vi "side_features.vi"() -> ()   [LabVIEW 2015]
uses:
  <vilib>/Analysis/baseanly.llb/Mean (DBL).vi
  <vilib>/Utility/file.llb/Read Delimited Spreadsheet (string).vi
  <vilib>/Utility/file.llb/Write Delimited Spreadsheet (string).vi
  <vilib>/vision/NI_Vision_Development_Module.lvlib
  PlantType.dll
  TotalContoursConvexHull.dll
  2-top_features_oilseed/HistProperty.dll
  <vilib>/Analysis/NI_AALBase.lvlib
panel:
  out "savePath":path
  out "appended array":string[](array[string])
  out "im_width":i32
  out "im_height":i32
  in  "Date Path":path=path "H:/3-side_features_oilseed/rape_test/path.txt"
  out "Current Path":path
  out "Current Number":string
  out "Rotated Image":T1(plugin-control)
  out "HistStat_whole":dbl[](array[numeric])
  out "PAR (perimeter-to-area ratio)":dbl
  out "SFD":sgl
  out "BW (minimum circumscribed box width)":dbl
  out "BH (minimum circumscribed box height)":dbl
  out "TPA (Total projective area)":dbl
  out "R (Rectangularity)":dbl
  out "IFD":sgl
  out "Hull area":dbl
  out "AC (Area Convexity)":dbl
  out "HWR":dbl
  in  "ROI_flower":T2={"Top"=0, "im_height"=1450, "L_left"=0, "im_width"=1680}
  out "NB (Number of blanchs)":i32
  out "FPAR (Flower perimeter-to-area ratio)":dbl
  out "FSFD":sgl
  out "FBW (Flower minimum circumscribed box width)":dbl
  out "FBH (Flower minimum circumscribed box height)":dbl
  out "YPA (Yellow projective area)":dbl
  out "FR (Flower rectangularity)":dbl
  out "FIFD":sgl
  out "FAC (Flower area Convexity)":dbl
  out "HistStat_flower":dbl[](array[numeric])
  in  "ROI_whole":T2={"Top"=90, "im_height"=1970, "L_left"=300, "im_width"=1450}
  out "FHWR":dbl
  out "GPA (Green projective area)":dbl
  out "GPAR (Green / Total)":dbl
  out "YPAR (Yellow / Total)":dbl
  out "Flower Hull Image":T1(plugin-control)
  out "Flower Hull Area":dbl
  out "Cropped Image":T1(plugin-control)
  out "Binary Image":T1(plugin-control)
  out "rgb Hull Image":T1(plugin-control)
  out "Flower Image (RGB)":T1(plugin-control)
  out "Flower Image (Label)":T1(plugin-control)
  out "PD1-6":sgl[](array[numeric])
  out "f array":dbl[](array[numeric])
  out "Combined Image":T1(plugin-control)
  out "Image Path":path
  in  "Image Main Path":path=path "H:/3-side_features_oilseed/rape_test"
  # "Digital evaluation software for oilseed rape phenotype-related traits (side-view) v1.0"
  # "测量数据"
  # "Whole plant"
  # "均值"
  # "标准差"
  # "平滑度"
  # "三阶矩"
  # "一致性"
  # "熵"
  # "Flower"
  # "Ratio"
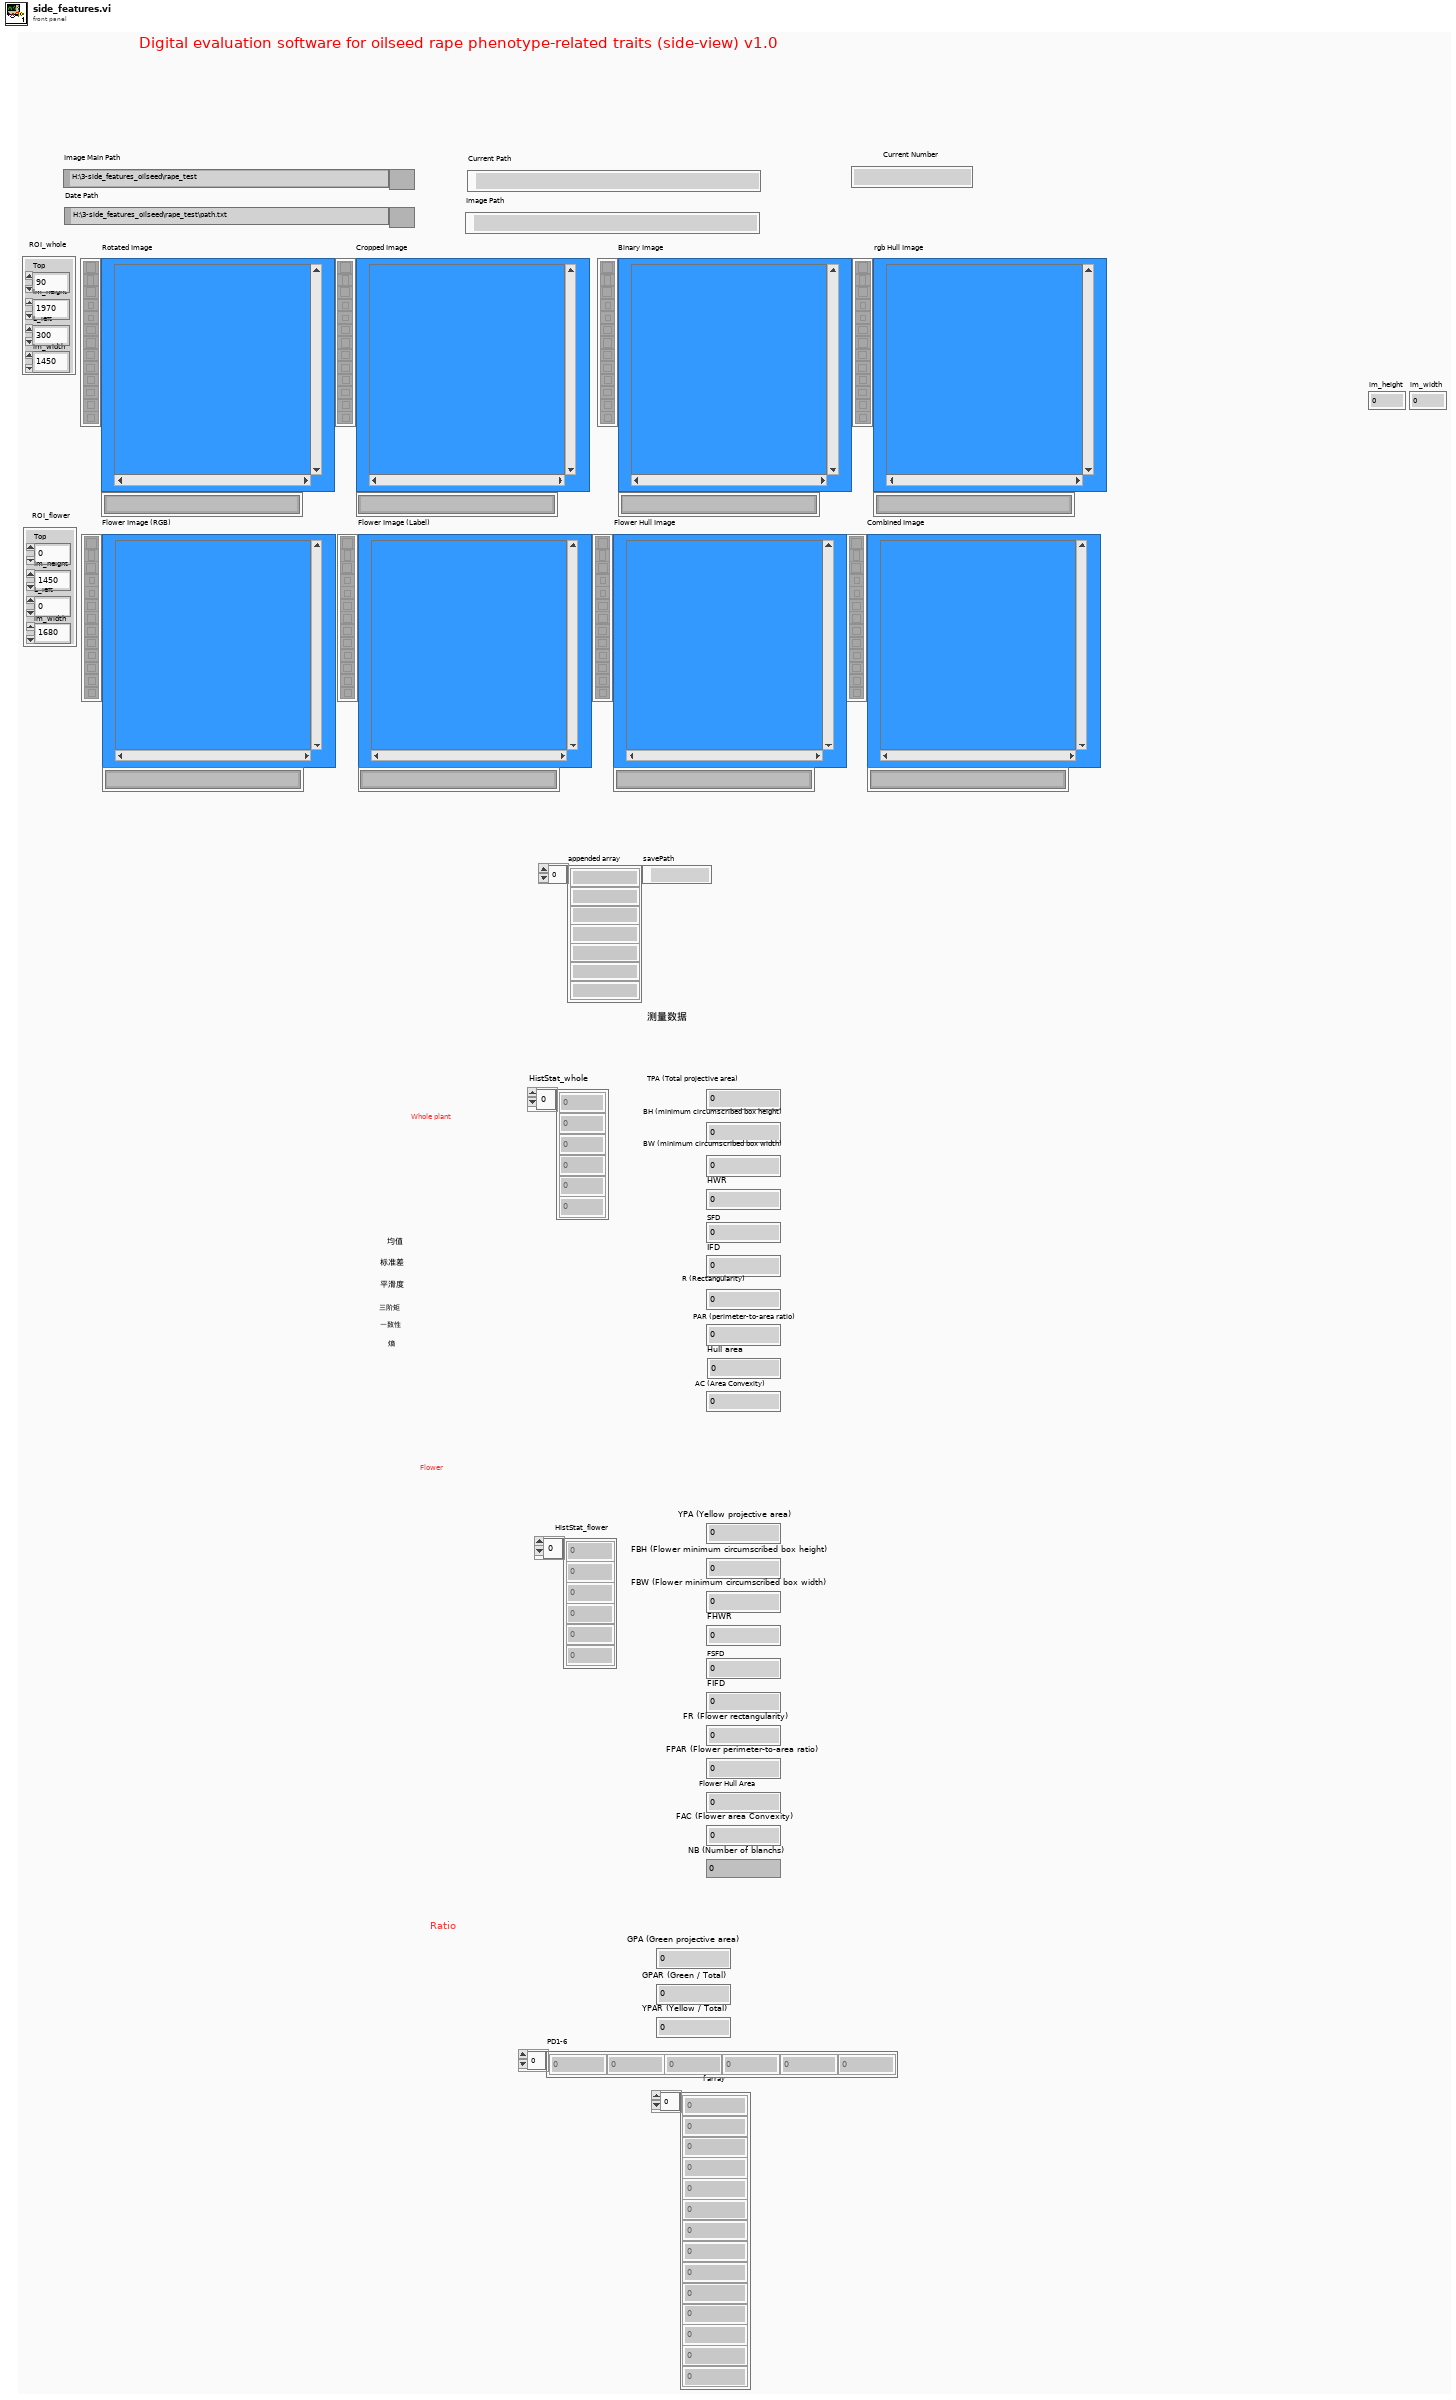
[diagram p1: front panel]
types:
  T1 = typedef "IMAQ Image.ctl" = refnum<image>
  T2 = cluster{"Top":i32, "im_height":i32, "L_left":i32, "im_width":i32}
  T3 = typedef "Image Type" = u32
  T4 = typedef "Particle Parameters" = i32
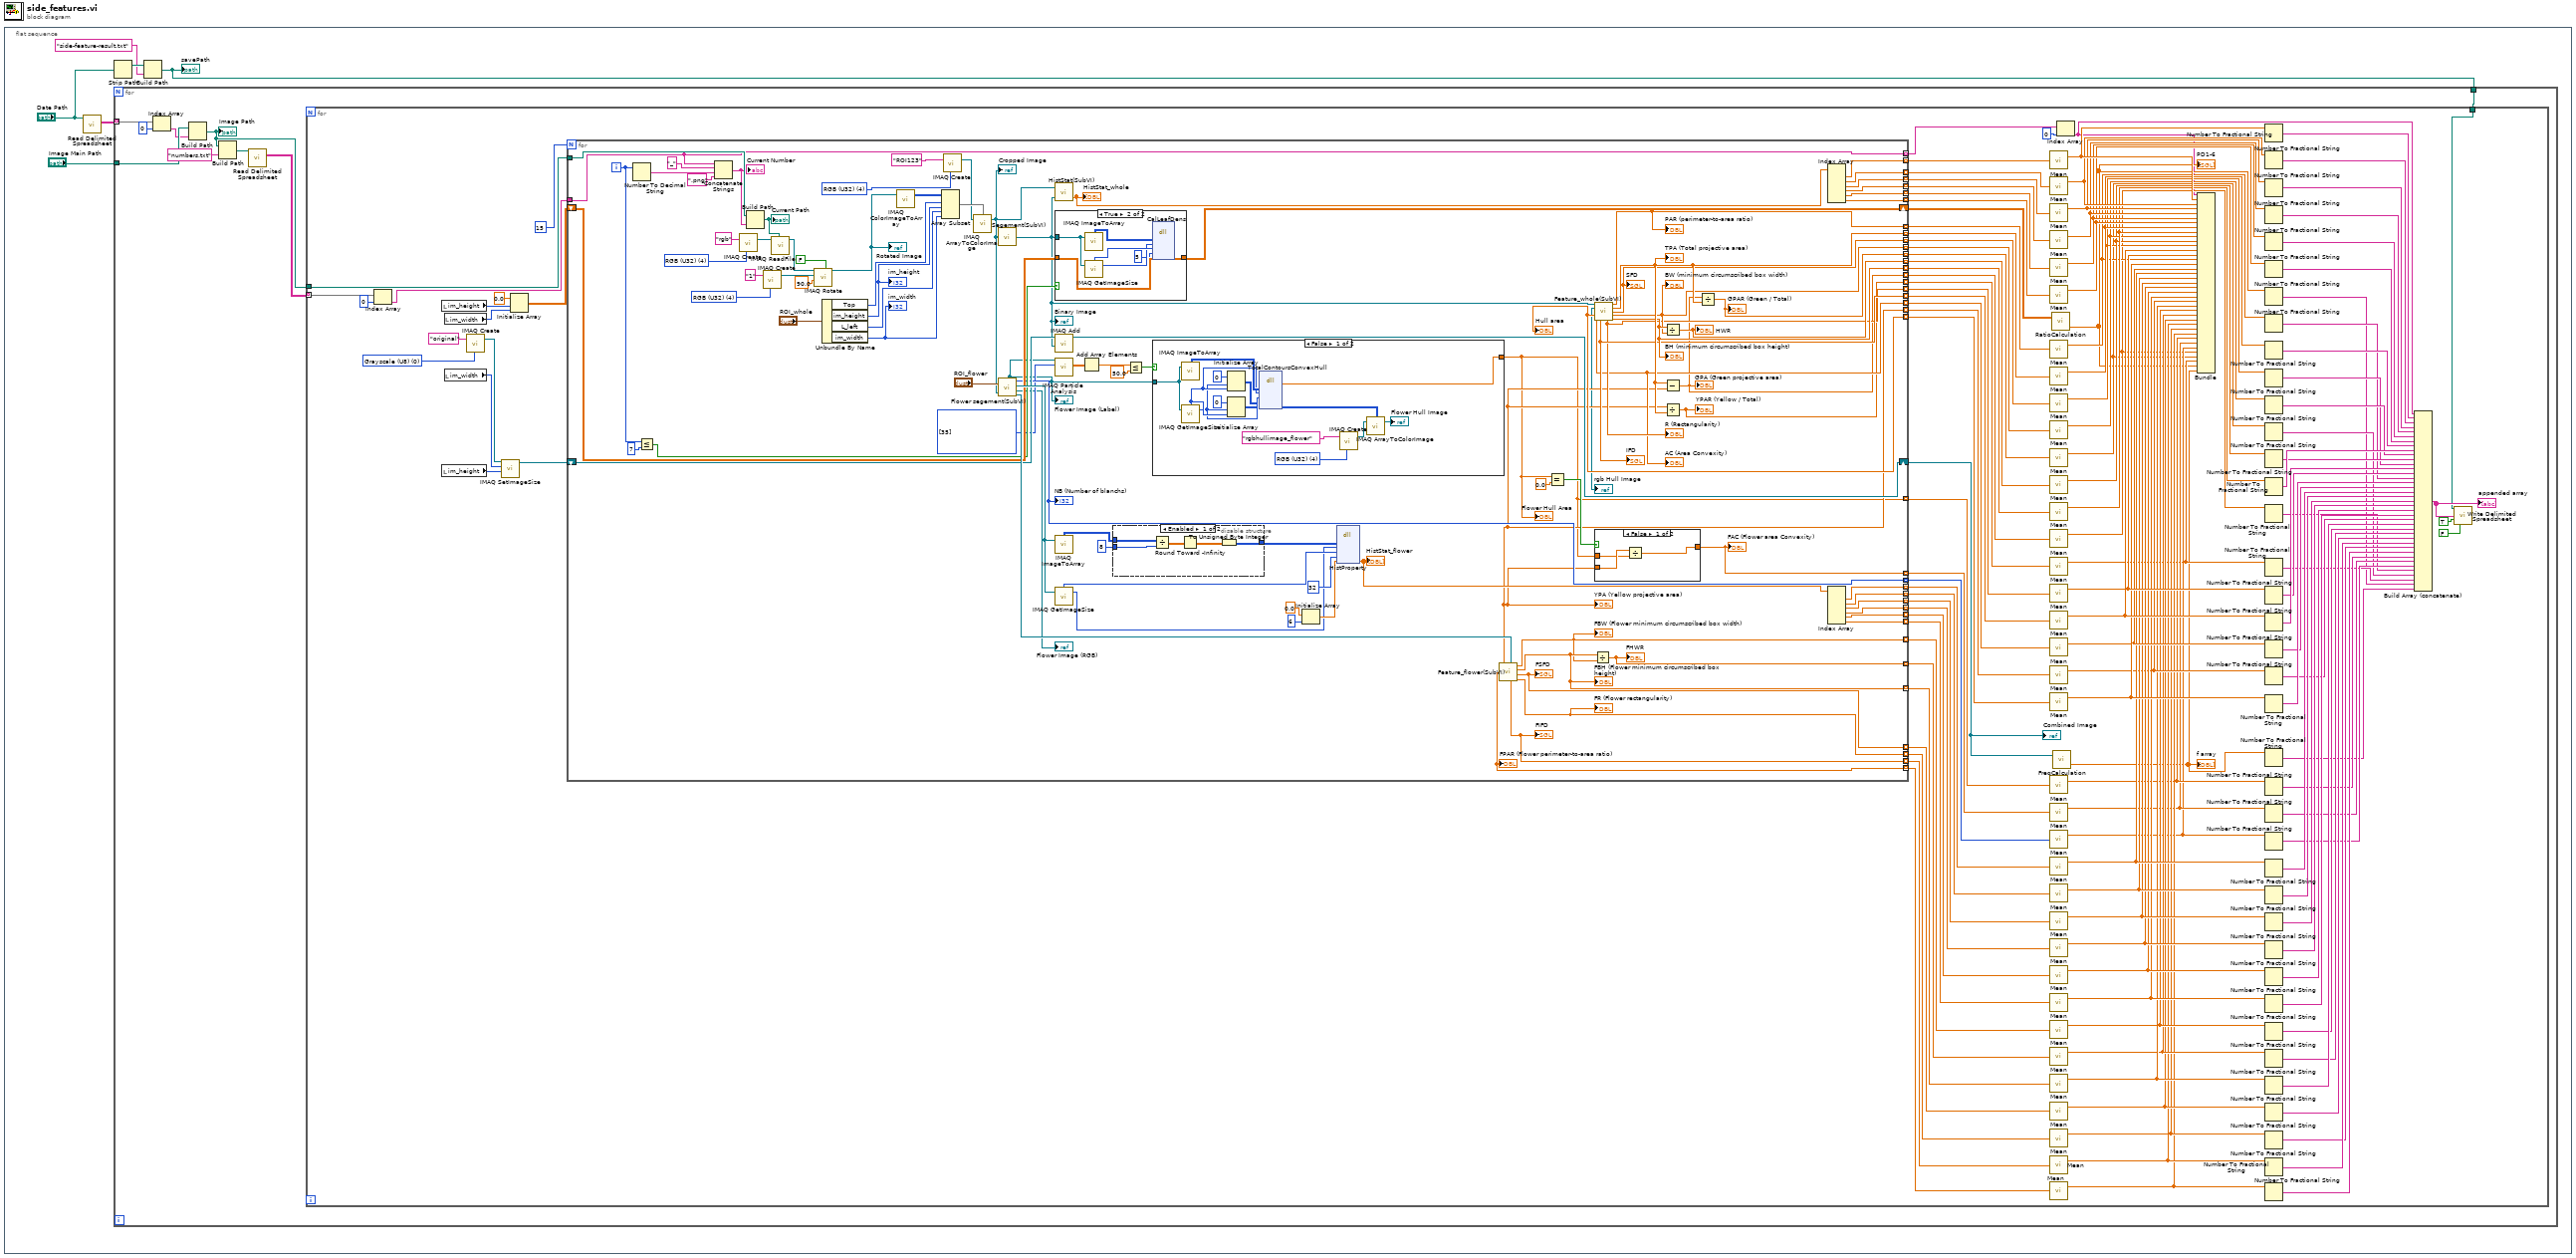
[diagram p0: block diagram]
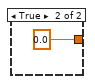
[diagram p2: hidden frame]
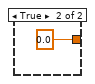
[diagram p3: hidden frame]
diagram:
  n1 = flat-sequence {
    frame #0 {
      n2 = call-poly <vilib>:"Read Delimited Spreadsheet.vi"("file path (dialog if empty)"="Date Path") -> ("all rows"=w5:string[][])  [unwired: 9 in, 5 out]
      n3 = Strip Path(path="Date Path") -> (stripped path=w3:path)  [unwired: 1 out]
      n4 = Build Path(base path=w3, name or relative path="side-feature-result.txt") -> (appended path=w1:path)
      "savePath" <- w1
      n5 = for {
        tunnel: "Image Main Path" -> [w15]
        tunnel: w5 -> [w13] mode=indexing
        tunnel: w1 -> [w7]
        n6 = Index Array(array=w13, index=0) -> (element=w9:string)
        n7 = Build Path(base path=w15, name or relative path=w9) -> (appended path=w10:path)
        "Image Path" <- w10
        n8 = Build Path(base path=w10, name or relative path="numbers.txt") -> (appended path=w11:path)
        n9 = call-poly <vilib>:"Read Delimited Spreadsheet.vi"("file path (dialog if empty)"=w11) -> ("all rows"=w8:string[][])  [unwired: 9 in, 5 out]
        n10 = for {
          tunnel: w10 -> [w149]
          tunnel: w8 -> [w150] mode=indexing
          tunnel: w7 -> [w16]
          w141 = T3 0 items=["Grayscale (U8)", "Grayscale (I16)", "Grayscale (SGL)", "Complex (CSG)", "RGB (U32)", "HSL (U32)", "RGB (U64)", "Grayscale (U16)"] ("Image Type")
          n11 = Index Array(array=w150, index=0) -> (element=w148:string)
          n12 = local read "im_height"() -> (w100:i32)
          n13 = local read "im_height"() -> (w99:i32)
          n14 = local read "im_width"() -> (w98:i32)
          n15 = local read "im_width"() -> (w97:i32)
          n16 = call "IMAQ Create"("Image Name"="original", "Image Type"=w141) -> ("New Image"=w142:T1)  [unwired: 2 in, 2 out]
          n17 = call "IMAQ SetImageSize"("Y Resolution"=w99, "X Resolution"=w97, "Image"=w142) -> ("Image Out"=w140:T1)  [unwired: 1 in, 2 out]
          n18 = Initialize Array(sgl 0.0 ("element"), w100, w98) -> (w145:sgl[][])
          n19 = for {
            N: 15 -> [_]
            tunnel: w149 -> [w240]
            tunnel: w148 -> [w153]
            shift-right: [w206] -> w144
            shift-left: w145 -> [w209]
            shift-right: [w204] -> w103
            shift-left: w140 -> [w205]
            tunnel: [w202] -> w139 mode=indexing
            tunnel: [w201] -> w138 mode=indexing
            tunnel: [w200] -> w137 mode=indexing
            tunnel: [w199] -> w136 mode=indexing
            tunnel: [w198] -> w135 mode=indexing
            tunnel: [w197] -> w134 mode=indexing
            tunnel: [w196] -> w133 mode=indexing
            tunnel: [w195] -> w132 mode=indexing
            tunnel: [w194] -> w131 mode=indexing
            tunnel: [w193] -> w130 mode=indexing
            tunnel: [w192] -> w129 mode=indexing
            tunnel: [w191] -> w128 mode=indexing
            tunnel: [w190] -> w127 mode=indexing
            tunnel: [w189] -> w126 mode=indexing
            tunnel: [w188] -> w125 mode=indexing
            tunnel: [w187] -> w124 mode=indexing
            tunnel: [w185] -> w123 mode=indexing
            tunnel: [w184] -> w122 mode=indexing
            tunnel: [w183] -> w121 mode=indexing
            tunnel: [w182] -> w120 mode=indexing
            tunnel: [w181] -> w119 mode=indexing
            tunnel: [w180] -> w118 mode=indexing
            tunnel: [w161] -> w117 mode=indexing
            tunnel: [w179] -> w116 mode=indexing
            tunnel: [w178] -> w115 mode=indexing
            tunnel: [w177] -> w114 mode=indexing
            tunnel: [w176] -> w113 mode=indexing
            tunnel: [w175] -> w112 mode=indexing
            tunnel: [w174] -> w111 mode=indexing
            tunnel: [w173] -> w110 mode=indexing
            tunnel: [w160] -> w109 mode=indexing
            tunnel: [w159] -> w108 mode=indexing
            tunnel: [w172] -> w107 mode=indexing
            tunnel: [w171] -> w106 mode=indexing
            tunnel: [w170] -> w105 mode=indexing
            tunnel: [w169] -> w104 mode=indexing
            tunnel: [w153] -> w102 mode=indexing
            i -> [w152]
            w168 = T4[] [35] items=["Center of Mass X", "Center of Mass Y", "First Pixel X", "First Pixel Y", "Bounding Rect Left", "Bounding Rect Top", "Bounding Rect Right", "Bounding Rect Bottom", "Max Feret Diameter Start X", "Max Feret Diameter Start Y", "Max Feret Diameter End X", "Max Feret Diameter End Y", "Max Horiz. Segment Length Left", "Max Horiz. Segment Length Right", "Max Horiz. Segment Length Row", "-", "Bounding Rect Width", "Bounding Rect Height", "Bounding Rect Diagonal", "Perimeter", "Convex Hull Perimeter", "Holes' Perimeter", "Max Feret Diameter", "Equivalent Ellipse Major Axis", "Equivalent Ellipse Minor Axis", "Equivalent Ellipse Minor Axis (Feret)", "Equivalent Rect Long Side", "Equivalent Rect Short Side", "Equivalent Rect Diagonal", "Equivalent Rect Short Side (Feret)", "Average Horiz. Segment Length", "Average Vert. Segment Length", "Hydraulic Radius", "Waddel Disk Diameter", "-", "Area", "Holes' Area", "Particle & Holes' Area", "Convex Hull Area", "Image Area", "-", "Number of Holes", "Number of Horiz. Segments", "Number of Vert. Segments", "-", "Orientation", "Max Feret Diameter Orientation", "-", "% Area/Image Area", "% Area/(Particle & Holes' Area)", "Ratio of Equivalent Ellipse Axes", "Ratio of Equivalent Rect Sides", "-", "Elongation Factor", "Compactness Factor", "Heywood Circularity Factor", "Type Factor", "-", "Sum X", "Sum Y", "Sum XX", "Sum XY", "Sum YY", "Sum XXX", "Sum XXY", "Sum XYY", "Sum YYY", "-", "Moment of Inertia XX", "Moment of Inertia XY", "Moment of Inertia YY", "Moment of Inertia XXX", "Moment of Inertia XXY", "Moment of Inertia XYY", "Moment of Inertia YYY", "Norm. Moment of Inertia XX", "Norm. Moment of Inertia XY", "Norm. Moment of Inertia YY", "Norm. Moment of Inertia XXX", "Norm. Moment of Inertia XXY", "Norm. Moment of Inertia XYY", "Norm. Moment of Inertia YYY", "Hu Moment 1", "Hu Moment 2", "Hu Moment 3", "Hu Moment 4", "Hu Moment 5", "Hu Moment 6", "Hu Moment 7"] ("Pixel Measurements")
            w225 = u32 4 items=["Grayscale (U8)", "Grayscale (I16)", "Grayscale (SGL)", "Complex (CSG)", "RGB (U32)", "HSL (U32)", "RGB (U64)"] ("Image Type")
            w238 = T3 4 items=["Grayscale (U8)", "Grayscale (I16)", "Grayscale (SGL)", "Complex (CSG)", "RGB (U32)", "HSL (U32)", "RGB (U64)", "Grayscale (U16)"] ("Image Type")
            w245 = T3 4 items=["Grayscale (U8)", "Grayscale (I16)", "Grayscale (SGL)", "Complex (CSG)", "RGB (U32)", "HSL (U32)", "RGB (U64)", "Grayscale (U16)"] ("Image Type")
            n20 = Number To Decimal String(number=w152) -> (decimal integer string=w242:string)  [unwired: 1 out]
            n21 = Less Or Equal?(x=w152, y=u32 7) -> (x <= y?=w207:bool)
            n22 = Concatenate Strings(w153, "_" ("string"), w242, ".png" ("string")) -> (w234:string)
            "Current Number" <- w234
            n23 = call "IMAQ Create"("Image Name"="rgb", "Image Type"=w245) -> ("New Image"=w246:T1)  [unwired: 2 in, 2 out]
            n24 = Build Path(base path=w240, name or relative path=w234) -> (appended path=w241:path)
            "Current Path" <- w241
            n25 = call "IMAQ Create"("Image Name"="1", "Image Type"=w238) -> ("New Image"=w236:T1)  [unwired: 2 in, 2 out]
            n26 = call "IMAQ ReadFile"("File Path"=w241, "Image"=w246) -> ("Image Out"=w233:T1)  [unwired: 3 in, 6 out]
            n27 = call "IMAQ Rotate"("Maintain Size"=FALSE, "Angle (degrees)"=sgl 90.0, "Image Dst"=w236, "Image Src"=w233) -> ("Image Dst Out"=w223:T1)  [unwired: 4 in, 3 out]
            "Rotated Image" <- w223
            n28 = Unbundle By Name("ROI_whole") -> ("Top"=w229:i32, "im_height"=w230:i32, "L_left"=w231:i32, "im_width"=w232:i32)
            "im_height" <- w230
            "im_width" <- w232
            n29 = call "IMAQ ColorImageToArray"("Image"=w223) -> ("Image Pixels (U32)"=w228:u32[][])  [unwired: 2 in, 3 out]
            n30 = Array Subset(array=w228, index (row)=w229, length (row)=w230, index (col)=w231, length (col)=w232) -> (w227:u32[][])
            n31 = call "IMAQ Create"("Image Name"="ROI123", "Image Type"=w225) -> ("New Image"=w224:T1)  [unwired: 2 in, 2 out]
            n32 = call "IMAQ ArrayToColorImage"("Image Pixels (U32)"=w227, "Image"=w224) -> ("Image Out"=w158:T1)  [unwired: 2 in, 2 out]
            "Cropped Image" <- w158
            n33 = call "Segement(SubVI).vi"("Image in"=w158) -> ("Binary Image"=w157:T1)
            "Binary Image" <- w157
            n34 = call "Flower segement(SubVI).vi"("Image in"=w158, "ROI 上半部分 2"="ROI_flower") -> ("黄色分量（油菜花）二值图"=w221:T1, "黄色分量（油菜花）"=→"Flower Image (RGB)":T1, "黄色分量（油菜花）Gray"=w211:T1, "Number of Particles"=w172:i32, "RGB花标记"=w154:T1)
            "NB (Number of blanchs)" <- w172
            "Flower Image (Label)" <- w154
            n35 = call "HistStat(SubVI).vi"("Binary Image"=w157, "Original Image"=w158) -> ("HistStat"=w203:dbl[])  [unwired: 1 out]
            "HistStat_whole" <- w203
            n36 = case shown="True" w207 {
              tunnel: w157 -> [_ w271]
              tunnel: w209 -> [w267 w270]
              tunnel: [w267 w269] -> w206
              frame False {
              }
              frame True {
                n37 = call "IMAQ ImageToArray"("Image"=w271) -> ("Image Pixels (U8)"=w274:u8[][])  [unwired: 2 in, 5 out]
                n38 = call "IMAQ GetImageSize"("Image"=w271) -> ("Y Resolution"=w272:i32, "X Resolution"=w273:i32)  [unwired: 1 in, 3 out]
                n39 = dll-call lib="H:/3-side_features_oilseed/PlantType.dll" fn="CalLeafDens"("bw"=w274, "row"=w272, "col"=w273, "GridSize"=5, "dens"=w270) -> ("dens"=w269:sgl[][])  [unwired: 7 in, 3 out]
              }
            }
            n40 = call "IMAQ Add"("Image Src A"=w205, "Image Src B"=w157) -> ("Image Dst Out"=w204:T1)  [unwired: 3 in, 3 out]
            n41 = call "IMAQ Particle Analysis"("Pixel Measurements"=w168, "Image"=w154) -> ("Particle Measurements (Pixels)"=w167:dbl[][])  [unwired: 3 in, 6 out]
            n42 = call "IMAQ ImageToArray"("Image"=w211) -> ("Image Pixels (U8)"=w212:u8[][])  [unwired: 2 in, 5 out]
            n43 = call "IMAQ GetImageSize"("Image"=w211) -> ("Y Resolution"=w215:i32, "X Resolution"=w216:i32)  [unwired: 1 in, 3 out]
            n44 = Add Array Elements(numeric array=w167) -> (sum=w166:dbl)
            n45 = disable-structure shown="Enabled" {
              disable-tunnel: w212 -> [w279 w280]
              disable-tunnel: u8 8 ("y") -> [w278 _]
              disable-tunnel: [w275 w280] -> w214
              frame Enabled {
                n46 = Divide(x=w279, y=w278) -> (x/y=w277:dbl[][])
                n47 = Round Toward -Infinity(1:w277) -> (0:w276:dbl[][])
                n48 = To Unsigned Byte Integer(number=w276) -> (unsigned 8bit integer=w275:u8[][])
              }
              frame Disabled {
              }
            }
            n49 = Less Or Equal?(x=w166, y=50.0) -> (x <= y?=w164:bool)
            n50 = case shown="False" w164 {
              tunnel: w154 -> [w254 _]
              tunnel: [w253 0.0 ("areaSum")] -> w160
              frame False {
                w260 = T3 4 items=["Grayscale (U8)", "Grayscale (I16)", "Grayscale (SGL)", "Complex (CSG)", "RGB (U32)", "HSL (U32)", "RGB (U64)", "Grayscale (U16)"] ("Image Type")
                n51 = call "IMAQ ImageToArray"("Image"=w254) -> ("Image Pixels (U8)"=w265:u8[][])  [unwired: 2 in, 5 out]
                n52 = call "IMAQ GetImageSize"("Image"=w254) -> ("Y Resolution"=w263:i32, "X Resolution"=w264:i32)  [unwired: 1 in, 3 out]
                n53 = Initialize Array(u8 0 ("element"), w263, w264) -> (w255:u8[][])
                n54 = Initialize Array(u32 0 ("element"), w263, w264) -> (w258:u32[][])
                n55 = dll-call lib="H:/3-side_features_oilseed/TotalContoursConvexHull.dll" fn="TotalContoursConvexHull"("src"=w265, "width"=w264, "height"=w263, "bwhullimage"=w255, "rgbhullimage"=w258) -> ("areaSum"=w253:dbl, "rgbhullimage"=w261:u32[][])  [unwired: 7 in, 2 out]
                n56 = call "IMAQ Create"("Image Name"="rgbhullimage_flower", "Image Type"=w260) -> ("New Image"=w262:T1)  [unwired: 2 in, 2 out]
                n57 = call "IMAQ ArrayToColorImage"("Image Pixels (U32)"=w261, "Image"=w262) -> ("Image Out"=→"Flower Hull Image":T1)  [unwired: 2 in, 2 out]
              }
              frame True {
              }
            }
            "Flower Hull Area" <- w160
            n58 = Initialize Array(0.0 ("element"), 6 ("dimension size")) -> (w219:dbl[])
            n59 = dll-call lib="H:/2-top_features_oilseed/HistProperty.dll" fn="HistProperty"("Im"=w214, "row"=w215, "col"=w216, "G"=32, "HistStat"=w219) -> ("HistStat"=w186:dbl[])  [unwired: 7 in, 3 out]
            "HistStat_flower" <- w186
            n60 = call "Feature_flower(SubVI).vi"("黄色分量（油菜花）二值图"=w221) -> ("SF 3"=w174:dbl, "IFD 2"=w175:sgl, "SFD 2"=w176:sgl, "SH 2"=w179:dbl, "SW 2"=w178:dbl, "SE 2"=w173:dbl, "SA"=w161:dbl)  [unwired: 1 out]
            "FPAR (Flower perimeter-to-area ratio)" <- w173
            "FSFD" <- w176
            "FBW (Flower minimum circumscribed box width)" <- w178
            "FBH (Flower minimum circumscribed box height)" <- w179
            "YPA (Yellow projective area)" <- w161
            "FR (Flower rectangularity)" <- w174
            "FIFD" <- w175
            n61 = Equal?(x=w160, y=0.0) -> (x = y?=w163:bool)
            n62 = Divide(x=w179, y=w178) -> (x/y=w177:dbl)
            "FHWR" <- w177
            n63 = call "Feature_whole(SubVI).vi"("Binary Image"=w157) -> ("SE"=w189:dbl, "rgb Hull Image 2"=→"rgb Hull Image":T1, "SA"=w196:dbl, "SFD"=w192:sgl, "Hull area"=w188:dbl, "SW"=w194:dbl, "SF 2"=w187:dbl, "IFD"=w191:sgl, "SF"=w190:dbl, "SH"=w195:dbl)  [unwired: 5 out]
            "PAR (perimeter-to-area ratio)" <- w189
            "SFD" <- w192
            "BW (minimum circumscribed box width)" <- w194
            "BH (minimum circumscribed box height)" <- w195
            "TPA (Total projective area)" <- w196
            "R (Rectangularity)" <- w190
            "IFD" <- w191
            "Hull area" <- w188
            "AC (Area Convexity)" <- w187
            n64 = case shown="False" w163 {
              tunnel: w161 -> [w250 _]
              tunnel: w160 -> [w249 _]
              tunnel: [w248 0.0] -> w159
              frame False {
                n65 = Divide(x=w250, y=w249) -> (x/y=w248:dbl)
              }
              frame True {
              }
            }
            "FAC (Flower area Convexity)" <- w159
            n66 = Divide(x=w195, y=w194) -> (x/y=w193:dbl)
            "HWR" <- w193
            n67 = Subtract(x=w196, y=w161) -> (x-y=w171:dbl)
            "GPA (Green projective area)" <- w171
            n68 = Divide(x=w161, y=w196) -> (x/y=w169:dbl)
            "YPAR (Yellow / Total)" <- w169
            n69 = Divide(x=w171, y=w196) -> (x/y=w170:dbl)
            "GPAR (Green / Total)" <- w170
            n70 = Index Array(array=w203) -> (element #1=w202:dbl, element #2=w201:dbl, element #3=w200:dbl, element #4=w199:dbl, element #5=w198:dbl, element #6=w197:dbl)  [unwired: 6 in]
            n71 = Index Array(array=w186) -> (element #1=w185:dbl, element #2=w184:dbl, element #3=w183:dbl, element #4=w182:dbl, element #5=w181:dbl, element #6=w180:dbl)  [unwired: 6 in]
          }
          "Combined Image" <- w103
          n72 = call-poly <vilib>:"Mean.vi"("X"=w139) -> ("mean"=w96:dbl)  [unwired: 1 out]
          n73 = call-poly <vilib>:"Mean.vi"("X"=w138) -> ("mean"=w95:dbl)  [unwired: 1 out]
          n74 = call-poly <vilib>:"Mean.vi"("X"=w137) -> ("mean"=w94:dbl)  [unwired: 1 out]
          n75 = call-poly <vilib>:"Mean.vi"("X"=w136) -> ("mean"=w93:dbl)  [unwired: 1 out]
          n76 = call-poly <vilib>:"Mean.vi"("X"=w135) -> ("mean"=w92:dbl)  [unwired: 1 out]
          n77 = call-poly <vilib>:"Mean.vi"("X"=w134) -> ("mean"=w91:dbl)  [unwired: 1 out]
          n78 = call-poly <vilib>:"Mean.vi"("X"=w126) -> ("mean"=w83:dbl)  [unwired: 1 out]
          n79 = call-poly <vilib>:"Mean.vi"("X"=w133) -> ("mean"=w90:dbl)  [unwired: 1 out]
          n80 = call-poly <vilib>:"Mean.vi"("X"=w129) -> ("mean"=w86:dbl)  [unwired: 1 out]
          n81 = call-poly <vilib>:"Mean.vi"("X"=w131) -> ("mean"=w88:dbl)  [unwired: 1 out]
          n82 = call-poly <vilib>:"Mean.vi"("X"=w105) -> ("mean"=w62:dbl)  [unwired: 1 out]
          n83 = call-poly <vilib>:"Mean.vi"("X"=w130) -> ("mean"=w87:dbl)  [unwired: 1 out]
          n84 = call-poly <vilib>:"Mean.vi"("X"=w132) -> ("mean"=w89:dbl)  [unwired: 1 out]
          n85 = call-poly <vilib>:"Mean.vi"("X"=w106) -> ("mean"=w63:dbl)  [unwired: 1 out]
          n86 = call-poly <vilib>:"Mean.vi"("X"=w104) -> ("mean"=w61:dbl)  [unwired: 1 out]
          n87 = call-poly <vilib>:"Mean.vi"("X"=w127) -> ("mean"=w84:dbl)  [unwired: 1 out]
          n88 = call-poly <vilib>:"Mean.vi"("X"=w128) -> ("mean"=w85:dbl)  [unwired: 1 out]
          n89 = call-poly <vilib>:"Mean.vi"("X"=w124) -> ("mean"=w81:dbl)  [unwired: 1 out]
          n90 = call-poly <vilib>:"Mean.vi"("X"=w117) -> ("mean"=w74:dbl)  [unwired: 1 out]
          n91 = call-poly <vilib>:"Mean.vi"("X"=w125) -> ("mean"=w82:dbl)  [unwired: 1 out]
          n92 = call-poly <vilib>:"Mean.vi"("X"=w109) -> ("mean"=w66:dbl)  [unwired: 1 out]
          n93 = call-poly <vilib>:"Mean.vi"("X"=w108) -> ("mean"=w65:dbl)  [unwired: 1 out]
          n94 = call-poly <vilib>:"Mean.vi"("X"=w107) -> ("mean"=w64:dbl)  [unwired: 1 out]
          n95 = call-poly <vilib>:"Mean.vi"("X"=w123) -> ("mean"=w80:dbl)  [unwired: 1 out]
          n96 = call-poly <vilib>:"Mean.vi"("X"=w122) -> ("mean"=w79:dbl)  [unwired: 1 out]
          n97 = call-poly <vilib>:"Mean.vi"("X"=w121) -> ("mean"=w78:dbl)  [unwired: 1 out]
          n98 = call-poly <vilib>:"Mean.vi"("X"=w120) -> ("mean"=w77:dbl)  [unwired: 1 out]
          n99 = call-poly <vilib>:"Mean.vi"("X"=w119) -> ("mean"=w76:dbl)  [unwired: 1 out]
          n100 = call-poly <vilib>:"Mean.vi"("X"=w118) -> ("mean"=w75:dbl)  [unwired: 1 out]
          n101 = call-poly <vilib>:"Mean.vi"("X"=w115) -> ("mean"=w72:dbl)  [unwired: 1 out]
          n102 = call-poly <vilib>:"Mean.vi"("X"=w114) -> ("mean"=w71:dbl)  [unwired: 1 out]
          n103 = call-poly <vilib>:"Mean.vi"("X"=w116) -> ("mean"=w73:dbl)  [unwired: 1 out]
          n104 = call-poly <vilib>:"Mean.vi"("X"=w113) -> ("mean"=w70:dbl)  [unwired: 1 out]
          n105 = call-poly <vilib>:"Mean.vi"("X"=w111) -> ("mean"=w68:dbl)  [unwired: 1 out]
          n106 = call-poly <vilib>:"Mean.vi"("X"=w112) -> ("mean"=w69:dbl)  [unwired: 1 out]
          n107 = call-poly <vilib>:"Mean.vi"("X"=w110) -> ("mean"=w67:dbl)  [unwired: 1 out]
          n108 = call "RatioCalculation.vi"("dens"=w144) -> ("ratio"=w60:sgl[])  [unwired: 2 out]
          "PD1-6" <- w60
          n109 = call "FreqCalculation.vi"("Acc Image"=w103) -> ("f array"=w59:dbl[])  [unwired: 2 out]
          "f array" <- w59
          n110 = Index Array(array=w102, index=0) -> (element=w24:string)
          n111 = Bundle("String"=w24, "mean"=w96, "mean"=w95, "mean"=w94, "mean"=w93, "mean"=w92, "mean"=w91, "mean"=w90, "mean"=w89, "mean"=w88, "mean"=w87, "mean"=w86, "mean"=w85, "mean"=w84, "mean"=w83, "mean"=w82, "mean"=w81, "mean"=w80, "mean"=w79, "mean"=w78, "mean"=w77, "mean"=w76, "mean"=w75, "mean"=w74, "mean"=w73, "mean"=w72, "mean"=w71, "mean"=w70, "mean"=w69, "mean"=w68, "mean"=w67, "mean"=w66, "mean"=w65, "mean"=w64, "mean"=w63, "mean"=w62, "mean"=w61, "ratio"=w60, "f array"=w59) -> ()  [unwired: 1 in, 1 out]
          n112 = Number To Fractional String(number=w96) -> (F-format string=w23:string)  [unwired: 3 in]
          n113 = Number To Fractional String(number=w95) -> (F-format string=w22:string)  [unwired: 3 in]
          n114 = Number To Fractional String(number=w94) -> (F-format string=w21:string)  [unwired: 3 in]
          n115 = Number To Fractional String(number=w93) -> (F-format string=w20:string)  [unwired: 3 in]
          n116 = Number To Fractional String(number=w92) -> (F-format string=w58:string)  [unwired: 3 in]
          n117 = Number To Fractional String(number=w91) -> (F-format string=w57:string)  [unwired: 3 in]
          n118 = Number To Fractional String(number=w60) -> (F-format string=w26:string[])  [unwired: 3 in]
          n119 = Number To Fractional String(number=w83) -> (F-format string=w49:string)  [unwired: 3 in]
          n120 = Number To Fractional String(number=w90) -> (F-format string=w56:string)  [unwired: 3 in]
          n121 = Number To Fractional String(number=w86) -> (F-format string=w52:string)  [unwired: 3 in]
          n122 = Number To Fractional String(number=w88) -> (F-format string=w54:string)  [unwired: 3 in]
          n123 = Number To Fractional String(number=w62) -> (F-format string=w28:string)  [unwired: 3 in]
          n124 = Number To Fractional String(number=w87) -> (F-format string=w53:string)  [unwired: 3 in]
          n125 = Number To Fractional String(number=w89) -> (F-format string=w55:string)  [unwired: 3 in]
          n126 = Number To Fractional String(number=w63) -> (F-format string=w29:string)  [unwired: 3 in]
          n127 = Number To Fractional String(number=w61) -> (F-format string=w27:string)  [unwired: 3 in]
          n128 = Number To Fractional String(number=w84) -> (F-format string=w50:string)  [unwired: 3 in]
          n129 = Number To Fractional String(number=w85) -> (F-format string=w51:string)  [unwired: 3 in]
          n130 = Number To Fractional String(number=w81) -> (F-format string=w47:string)  [unwired: 3 in]
          n131 = Number To Fractional String(number=w74) -> (F-format string=w40:string)  [unwired: 3 in]
          n132 = Number To Fractional String(number=w82) -> (F-format string=w48:string)  [unwired: 3 in]
          n133 = Number To Fractional String(number=w59) -> (F-format string=w25:string[])  [unwired: 3 in]
          n134 = Number To Fractional String(number=w66) -> (F-format string=w32:string)  [unwired: 3 in]
          n135 = Number To Fractional String(number=w65) -> (F-format string=w31:string)  [unwired: 3 in]
          n136 = Number To Fractional String(number=w64) -> (F-format string=w30:string)  [unwired: 3 in]
          n137 = Number To Fractional String(number=w80) -> (F-format string=w46:string)  [unwired: 3 in]
          n138 = Number To Fractional String(number=w79) -> (F-format string=w45:string)  [unwired: 3 in]
          n139 = Number To Fractional String(number=w78) -> (F-format string=w44:string)  [unwired: 3 in]
          n140 = Number To Fractional String(number=w77) -> (F-format string=w43:string)  [unwired: 3 in]
          n141 = Number To Fractional String(number=w76) -> (F-format string=w42:string)  [unwired: 3 in]
          n142 = Number To Fractional String(number=w75) -> (F-format string=w41:string)  [unwired: 3 in]
          n143 = Number To Fractional String(number=w72) -> (F-format string=w38:string)  [unwired: 3 in]
          n144 = Number To Fractional String(number=w71) -> (F-format string=w37:string)  [unwired: 3 in]
          n145 = Number To Fractional String(number=w73) -> (F-format string=w39:string)  [unwired: 3 in]
          n146 = Number To Fractional String(number=w70) -> (F-format string=w36:string)  [unwired: 3 in]
          n147 = Number To Fractional String(number=w68) -> (F-format string=w34:string)  [unwired: 3 in]
          n148 = Number To Fractional String(number=w69) -> (F-format string=w35:string)  [unwired: 3 in]
          n149 = Number To Fractional String(number=w67) -> (F-format string=w33:string)  [unwired: 3 in]
          n150 = Build Array (concatenate)(w24, w23, w22, w21, w20, w58, w57, w56, w55, w54, w53, w52, w51, w50, w49, w48, w47, w46, w45, w44, w43, w42, w41, w40, w39, w38, w37, w36, w35, w34, w33, w32, w31, w30, w29, w28, w27, w26, w25) -> (w19:string[])
          "appended array" <- w19
          n151 = call-poly <vilib>:"Write Delimited Spreadsheet.vi"("file path (dialog if empty)"=w16, "1D data"=w19, "append to file? (F)"=TRUE, "transpose? (F)"=FALSE) -> ()  [unwired: 10 in, 2 out]
        }
      }
    }
  }
